vi "RunDetection.vi"(4 "Specific target IP":string, 6 "Specific target (F)":bool, 7 "Reduce discovery timeout (T)":bool=TRUE, 8 "error in (no error)":errorcluster) -> (0 "error out":errorcluster, 3 "Filtered Targets":T1[](array[typedef]) {"IP Mode" items=["Static"=1, "DHCP/Link-Local"=2, "Link-Local Only"=4, "DHCP Only"=8]})   [LabVIEW 2013]
uses:
  types/MAX Sys Cfg Target Information.ctl
  globals/Globals.vi
  <vilib>/nisyscfg/Find Systems.vi
  <vilib>/nisyscfg/Close (System).vi
  <vilib>/nisyscfg/nisyscfg.lvlib
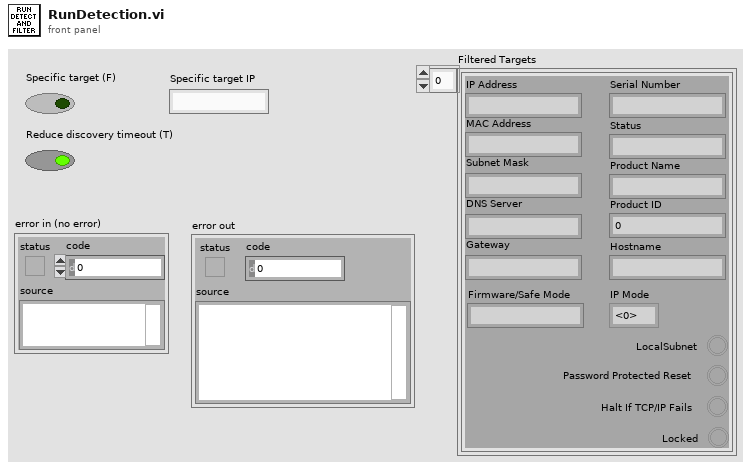
[diagram p1: front panel]
types:
  T1 = typedef "MAX Sys Cfg Target Information.ctl" = cluster{"MAC Address":string, "IP Address":string, "Status":string, "Product Name":string, "Hostname":string, "Firmware/Safe Mode":string, "Subnet Mask":string, "Gateway":string, "DNS Server":string, "Serial Number":string, "Product ID":u32, "Locked ":bool, "LocalSubnet":bool, "Halt If TCP/IP Fails":bool, "Password Protected Reset":bool, "IP Mode":i32}
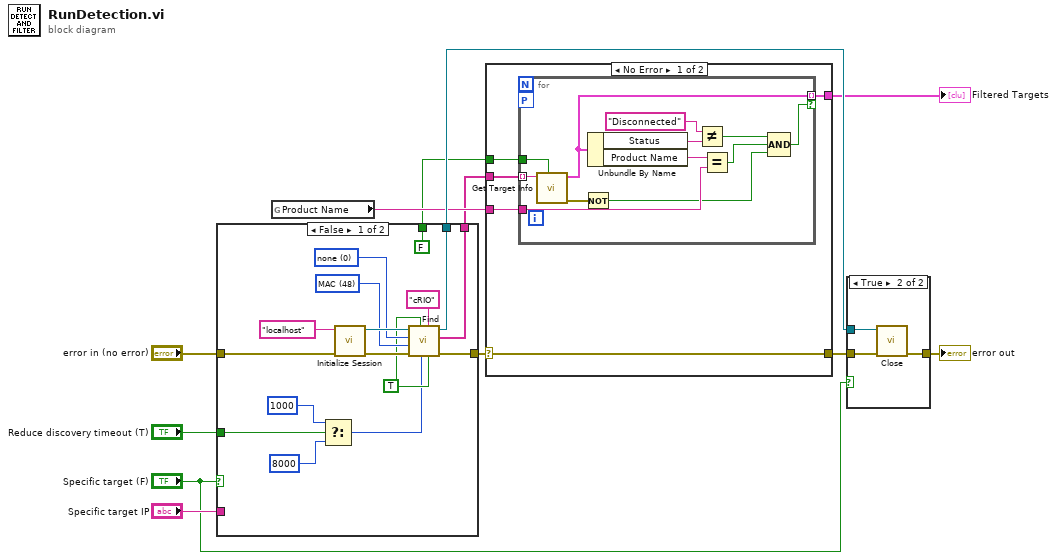
[diagram p0: block diagram]
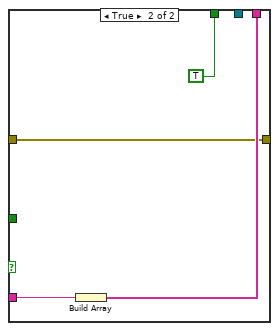
[diagram p3: hidden frame]
diagram:
  n1 = case shown="False" "Specific target (F)" {
    tunnel: "error in (no error)" -> [w28 w30]
    tunnel: [w25 _] -> w10
    tunnel: [w20 w30] -> w6
    tunnel: [w19 w31] -> w5
    tunnel: "Reduce discovery timeout (T)" -> [w17 _]
    tunnel: "Specific target IP" -> [_ w32]
    tunnel: [FALSE ("force property refresh (T)") TRUE ("force property refresh (T)")] -> w2
    frame False {
      w21 = TRUE ("only installable systems (F)")
      w23 = u32 48 items=["Hostname"=16, "Hostname (IP)"=18, "Hostname (MAC)"=19, "IP"=32, "IP (Hostname)"=33, "IP (MAC)"=35, "MAC"=48, "MAC (Hostname)"=49, "MAC (IP)"=50] ("output (hostname and IP)")
      w24 = u32 0 items=["none"=0, "only if online"=1, "all"=3] ("include cached results (all)")
      n2 = Select(t=u32 1000 ("timeout msec (4000)"), s=w17, f=u32 8000 ("timeout msec (4000)")) -> (s? t:f=w14:u32)
      n3 = call <vilib>:"Initialize Session.vi"("error in (no error)"=w28, "target (localhost)"="localhost") -> ("error out"=w27:errorcluster, "session out"=w26:refnum<k21>)  [unwired: 8 in]
      n4 = call-poly <vilib>:"Find.vi"("only installable systems (F)"=w21, "device class"="cRIO", "timeout msec (4000)"=w14, "detect online systems (T)"=w21, "error in (no error)"=w27, "output (hostname and IP)"=w23, "include cached results (all)"=w24, "session in (localhost)"=w26) -> ("error out"=w20:errorcluster, "detected systems"=w19:string[], "session out"=w25:refnum<k21>)  [unwired: 1 in]
    }
    frame True {
      n5 = Build Array(w32) -> (w31:string[])
    }
  }
  n6 = global read "Globals.vi" "Product Name"() -> (w9:string)
  n7 = case shown="No Error" w6 {
    selector: w6 -> [w35 w50]
    tunnel: w9 -> [w37 _]
    tunnel: [w36 _] -> w8
    tunnel: [w35 w50] -> w7
    tunnel: w5 -> [w34 _]
    tunnel: w2 -> [w33 _]
    frame No Error {
      n8 = for {
        tunnel: w37 -> [w49]
        tunnel: [w41] -> w36 mode=indexing if=w43
        workers-P: _ -> [_]
        tunnel: w34 -> [w39] mode=indexing
        tunnel: w33 -> [w38]
        n9 = call "Get Target Info.vi"("force property refresh (T)"=w38, "target"=w39) -> ("error out"=w40:errorcluster, "target info"=w41:T1)  [unwired: 8 in]
        n10 = Not(x=w40) -> (.not. x?=w42:bool)
        n11 = Unbundle By Name(w41) -> ("Status"=w47:string, "Product Name"=w48:string)
        n12 = Not Equal?(x="Disconnected", y=w47) -> (x != y?=w45:bool)
        n13 = Equal?(x=w48, y=w49) -> (x = y?=w44:bool)
        n14 = Compound Arithmetic op=AND(w45, w44, w42) -> (w43:bool)
      }
    }
    frame Error {
    }
  }
  "Filtered Targets" <- w8
  n15 = case shown="True" "Specific target (F)" {
    tunnel: [w51 w54] -> w11
    tunnel: w10 -> [_ w53]
    tunnel: w7 -> [w51 w52]
    frame False {
    }
    frame True {
      n16 = call-poly <vilib>:"Close.vi"("error in (no error)"=w52, "session in"=w53) -> ("error out"=w54:errorcluster)  [unwired: 9 in]
    }
  }
  "error out" <- w11
